vi "FRC ADI MXP IMU Example.vi"() -> ()   [LabVIEW 2015]
doc: "SimpleGyro Example\n\nThis example shows how to use a SimpleGyro sensor connected to the SPI port on the RoboRIO.\n\nThis example expects a USB cable connected from your development PC to the Type B USB Jack (next to the power input) on the roboRIO."
uses:
  <vilib>/Rock Robotics/SystemInterfaces/spilib/spi_bus.ctl
  ADI MXP IMU/FRC ADI MXP IMU.lvlib
panel:
  out "IMU AHRS":cluster{"Pitch":dbl, "Roll":dbl, "Yaw":dbl}
  out "IMU Data":T1
  out "IMU Angles":cluster{"X":dbl, "Y":dbl, "Z":dbl}
  in  "Reset Angles?":bool
  out "Device Found":bool
  in  "stop":bool
  in  "SPI Chip Select":T2=enum."SPI MXP"
  # "FRC Analog Devices IMU MXP Example"
  # "IMU Configuration \n(Can Only Be Changed at Start-Up)"
  # "FRC ADI MXP IMU Placement"
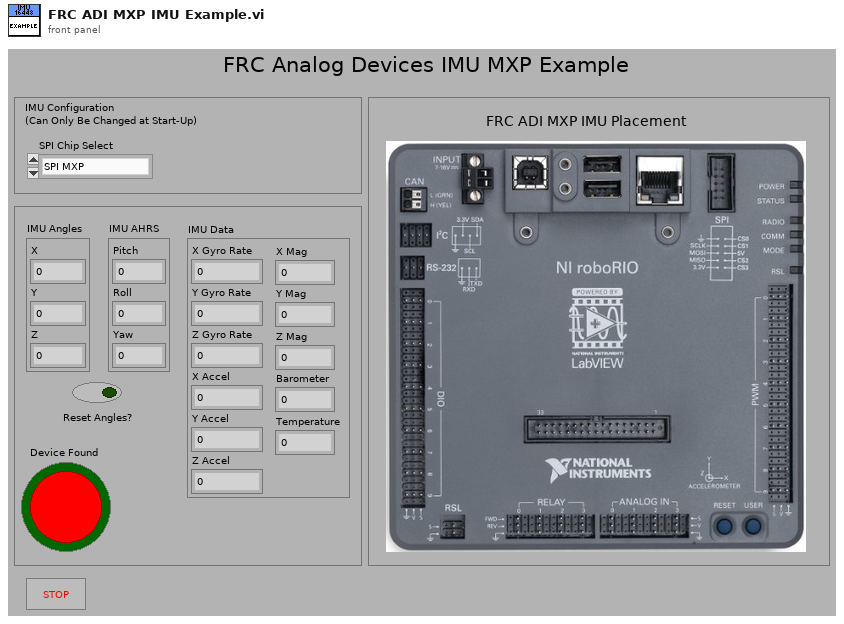
[diagram p1: front panel]
types:
  T1 = cluster{"X Gyro Rate":dbl, "Y Gyro Rate":dbl, "Z Gyro Rate":dbl, "X Accel":dbl, "Y Accel":dbl, "Z Accel":dbl, "X Mag":dbl, "Y Mag":dbl, "Z Mag":dbl, "Barometer":dbl, "Temperature":dbl}
  T2 = typedef "spi_bus.ctl" = enum16{"SPI On-Board, CS0", "SPI On-Board, CS1", "SPI On-Board, CS2", "SPI On-Board, CS3", "SPI MXP", "Invalid"}
  T3 = typedef "FRC ADI MXP IMU.lvlib/WPI_AnalogDevicesIMUDevRef.ctl" = cluster{"DevStatus":errorcluster, "Handle":i32, "SPI Bus":T2, "Device Found":bool, "Sample Rate":dbl}
  T4 = cluster{"X Angle":dbl, "Y Angle":dbl, "Z Angle":dbl}
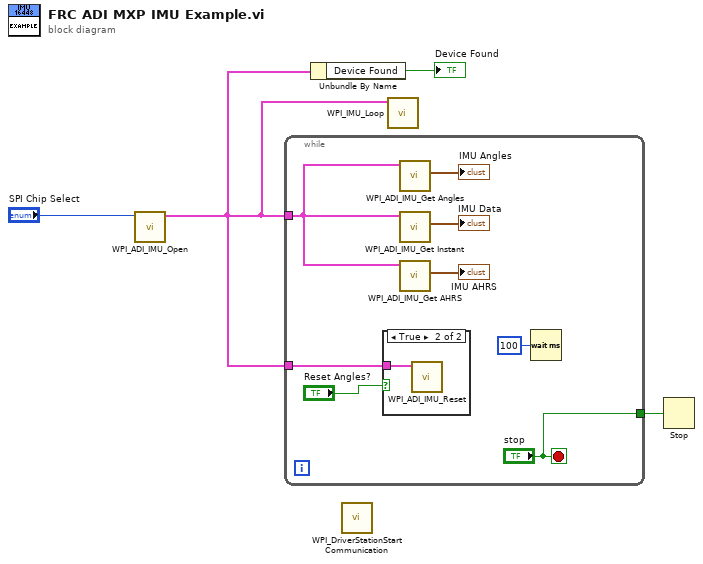
[diagram p0: block diagram]
diagram:
  n1 = call "WPI_ADI_IMU_Open.vi"("SPI Chip Select"="SPI Chip Select") -> ("IMUDevRef"=w1:T3)  [unwired: 9 in, 1 out]
  n2 = while {
    tunnel: w1 -> [w6]
    tunnel: ["stop"] -> w3
    tunnel: w1 -> [w10]
    stop <- "stop" stop-if-true
    n3 = case shown="True" "Reset Angles?" {
      tunnel: w10 -> [_ w13]
      frame False {
      }
      frame True {
        n4 = call "WPI_ADI_IMU_Reset.vi"("ADI IMU DevRef"=w13) -> ()  [unwired: 9 in, 2 out]
      }
    }
    n5 = call "WPI_ADI_IMU_Get Angles.vi"("ADIIMUDevRef"=w6) -> ("IMU Angles"=→"IMU Angles":T4)  [unwired: 8 in, 2 out]
    n6 = call "WPI_ADI_IMU_Get Instant.vi"("ADI IMU DevRef"=w6) -> ("IMU Data"=→"IMU Data":T1)  [unwired: 8 in, 2 out]
    n7 = call "WPI_ADI_IMU_Get AHRS.vi"("ADIIMUDevRef"=w6) -> ("IMU AHRS"=→"IMU AHRS":cluster{"Pitch":dbl, "Roll":dbl, "Yaw":dbl})  [unwired: 8 in, 2 out]
    n8 = Wait (ms)(milliseconds to wait=u32 100) -> ()  [unwired: 1 out]
  }
  n9 = Unbundle By Name(w1) -> ("Device Found"=→"Device Found":bool)
  n10 = call <vilib>:"WPI_DriverStationStart Communication.vi"() -> ()  [unwired: 12 in]
  n11 = call "WPI_IMU_Loop.vi"("SimpleGyroDevRef"=w1) -> ()  [unwired: 10 in, 1 out]
  n12 = Stop(stop? (T)=w3) -> ()
